vi "MrClean.destructor.vi"(0 "i ref in":refnum<vi>, 5 "error in(no error)":errorcluster) -> (19 "error out":errorcluster)   [LabVIEW 2014, in "MrClean.lvlib"]
doc: "This is the destructor of a class.\n\nLicense Agreement for this software:\n\nCopyright (C)\nGesellschaft für Schwerionenforschung, GSI\nPlanckstr. 1\n64291 Darmstadt\nGermany\n\nContact: D.Beck@gsi.de \n\nThis program is free software; you can redistribute it and/or modify it under the terms of the \nGNU General Public License as published by the Free Software Foundation; either version 2 of \nthe license, or (at your option) any later version.\n\nThis program is distributed in the hope that it will be useful, but WITHOUT ANY WARRANTY; \nwithout even the implied warranty of MERCHANTABILITY or FITNESS FOR A PARTICULAR PURPOSE. See the GNU General License for more details (http://www.gnu.org).\n\nGesellschaft für Schwerionenforschung, GSI\nPlanckstr. 1, 64291 Darmstadt, Germany\nFor all questions and ideas contact: M.Richter@gsi.de, H.Brand@gsi.de or D.Beck@gsi.de.\nLast update: 16-JUN-2004"
uses:
  MrClean.lvlib
  CS_Core/BaseProcess/BaseProcess.lvlib
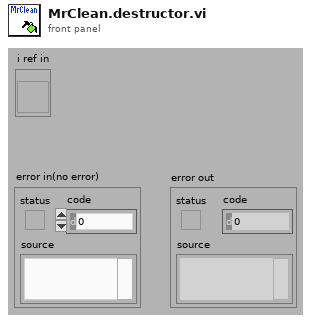
[diagram p1: front panel]
types:
  T1 = enum16{"SetAttribute", "GetAttribute", "CreateAttribute", "DestroyAttribute", "DestroyAllAtributes"}
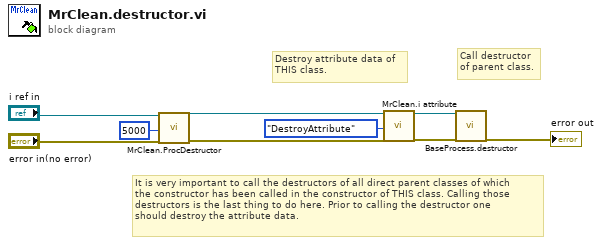
[diagram p0: block diagram]
diagram:
  # "It is very important to call the destructors of all direct parent classes of which\nthe constructor has been called in the constructor of THIS class. Calling those\ndestructors is the last thing to do here. Prior to calling the destructor one \nshould destroy the attribute data."
  # "Destroy attribute data of \nTHIS class."
  # "Call destructor\nof parent class."
  n1 = call "MrClean.ProcDestructor.vi"("i ref in"="i ref in", "ms timeout (100)"=5000, "error in (no error)"="error in(no error)") -> ("i ref out"=w5:refnum<vi>, "error out"=w1:errorcluster)  [unwired: 14 in, 1 out]
  n2 = call "MrClean.i attribute.vi"("VI Refnum"=w5, "Action"=T1."DestroyAttribute", "error in (no error)"=w1) -> ("VI Refnum out"=w8:refnum<vi>, "error out"=w7:errorcluster)  [unwired: 14 in, 1 out]
  n3 = call "BaseProcess.destructor.vi"("i ref in"=w8, "error in (no error)"=w7) -> ("error out"=→"error out":errorcluster)  [unwired: 17 in]
